vi "CRYSet Cell Value with Range.vi"(4 "Excel._Worksheet":refnum<k7>, 5 "error in (no error)":errorcluster, 6 "Value":string, 7 "Col":i32, 8 "Row":i32) -> (0 "error out":errorcluster, 1 "Cell":string, 2 "Range":refnum<k7>, 3 "Excel._Worksheet":refnum<k7>)   [LabVIEW 2013]
doc: "This VI sets the Value of the Cell in the WorkSheet designated by Row:Col to the input \"Value\". It first transforms the numeric row and column inputs to the Excel format of A1, B1 and so on. then it Executes the Range Method of the WorkSheet object and sets the \"Value\" property of the Range. It frees the automation Refnum of Range in each iteration of the loop."
panel:
  in  "dummy Range":refnum<k7>
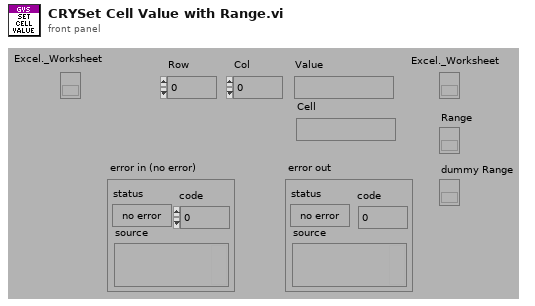
[diagram p1: front panel]
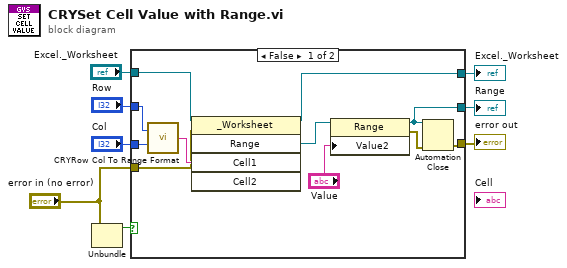
[diagram p0: block diagram]
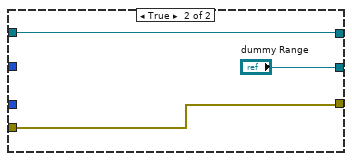
[diagram p2: hidden frame]
diagram:
  n1 = Unbundle("error in (no error)") -> ("status"=w4:bool)  [unwired: 2 out]
  n2 = case shown="False" w4 {
    tunnel: "Col" -> [w19 _]
    tunnel: "Row" -> [w18 _]
    tunnel: "error in (no error)" -> [w10 w22]
    tunnel: [w13 w22] -> w6
    tunnel: [w9 w21] -> w3
    tunnel: "Excel._Worksheet" -> [w12 w21]
    tunnel: [w11 "dummy Range"] -> w1
    frame False {
      n3 = call "CRYRow Col To Range Format.vi"("Column"=w19, "Row"=w18) -> ("Output String"=w17:string)
      n4 = invoke class="_Worksheet" method="Range"(reference=w12, error in=w10, "Cell1"=w17) -> (reference out=w9:refnum<k7>, "Range"=w16:refnum<k7>)  [unwired: 2 in, 3 out]
      n5 = property class="Range"(reference=w16, "Value2"="Value") -> (reference out=w11:refnum<k7>, error out=w14:errorcluster)  [unwired: 1 in]
      n6 = Automation Close(3:w14, 5:w11) -> (0:w13:errorcluster)
    }
    frame True {
    }
  }
  "Excel._Worksheet" <- w3
  "error out" <- w6
  "Range" <- w1
